vi "sv_Get X-Dimension String.vi"(4 "x-axis units":T1 items=["Time (s)"=0, "Frequency-CB (Hz)"=1, "Frequency-CPB (Hz)"=1248, "Frequency-Arbitrary (Hz)"=2357, "Quefrency (s)"=2, "Revolutions (rev)"=3, "Order"=4, "Speed (RPM)"=11, "Speed (rad/s)"=21, "Critical Band"=31, "Critical Band Rate (Bark)"=32, "None"=98, "Index"=65535]) -> (1 "x-domain string":string)   [LabVIEW 2017]
uses:
  <vilib>/addons/_NISVFA/_Shared subVIs/Controls/svc_X-Axis Units.ctl
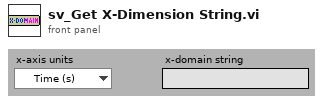
[diagram p1: front panel]
types:
  T1 = typedef "svc_X-Axis Units.ctl" = u16
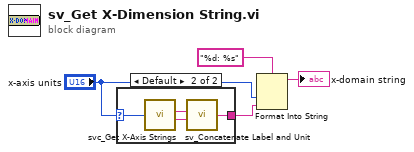
[diagram p0: block diagram]
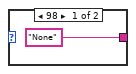
[diagram p2: hidden frame]
diagram:
  n1 = case shown="Default" "x-axis units" {
    selector: "x-axis units" -> [_ w6]
    tunnel: ["None" ("t") w7] -> w1
    frame 98 {
    }
    frame Default {
      n2 = call <vilib>:"svc_Get X-Axis Strings.vi"("x-axis units"=w6) -> ("x-axis label"=w8:string, "x-axis unit string"=w9:string)  [unwired: 4 in]
      n3 = call <vilib>:"sv_Concatenate Label and Unit.vi"("unit string"=w9, "label"=w8) -> ("scale label with units"=w7:string)  [unwired: 4 in]
    }
  }
  n4 = Format Into String(format string="%d: %s", "x-axis units", w1) -> (resulting string=→"x-domain string":string)  [unwired: 2 in, 1 out]
